vi "4_Generate_pulse_on_multiple channels.vi"() -> ()   [LabVIEW 2014]
uses:
  <vilib>/Swabian Instruments/Pulse Streamer/PulseStreamer/PulseStreamer/typedefs/typedef_TriggerStart.ctl
  <vilib>/Swabian Instruments/Pulse Streamer/PulseStreamer/PulsePattern/PulsePattern.lvclass
  <vilib>/Swabian Instruments/Pulse Streamer/PulseStreamer/typedefs/typedef_ChannelNumber.ctl
  <vilib>/Swabian Instruments/Pulse Streamer/PulseStreamer/Sequence/Sequence.lvclass
  <vilib>/Swabian Instruments/Pulse Streamer/PulseStreamer/PulseStreamer/stream/stream (Sequence).vi
  <vilib>/Swabian Instruments/Pulse Streamer/PulseStreamer/PulseStreamer/PulseStreamer.lvclass
  <vilib>/Swabian Instruments/Pulse Streamer/PulseStreamer/PulseStreamer.lvlib
panel:
  in  "nRuns":i64=1
  in  "ip or hostname":string="pulsestreamer"
  in  "Duration LOW":i64=1000
  out "error out":errorcluster
  in  "Repeat":u32=3
  in  "Start Type":T1
  in  "Duration HIGH":i64=500
  # "This example demonstrates how to generate synchronous signals on multiple channels.\n\nThe generated sequence consists of a square pulse on output channel \"0\" and three consecutive pulses on channels \"1\" and \"2\". \nThe pulses on channels \"1\" and \"2\" start on the falling edge of the pulse on channel \"0\".\n\nThis pulse sequence can be repeated finite or infinite number of times by specifying value of \"nRuns\".\nThe durations of each pulse are automatically split so that the Generated sequence has the Run Length Encoding (RLE)."
  # "PULSE DEFINITION"
  # "Every sequence has a repeat counter which can be used to repeat a\nsequence 'Repeat' times. \nIf there is only one sequence 'nRuns' from the 'stream' method should\nbe always used, because with 'Repeat' the data transferred to the \nPulsestreamer is repeated 'Repeat' times whereas nRuns sends the sequence\nonly once.\nRepeat >1 should be used when several sequences are combined and \neach sequence needs to be repeated."
  # "'nRuns' defines how many time the sequence has to be repeated by hardware\nnRuns<0 means that sequence will be repeated indefinitely"
  # "Defines whether the sequence starts \n* immediatly after it was uploaded  (IMMEDIATE)\n* after a software trigger (startNow) has been sent (SOFTWARE)\n* with an external trigger signal to \"Trigger\" input on the corresponding edge (HW_RISING, HW_FALLING, HW_RISING_AND_FALLING)."
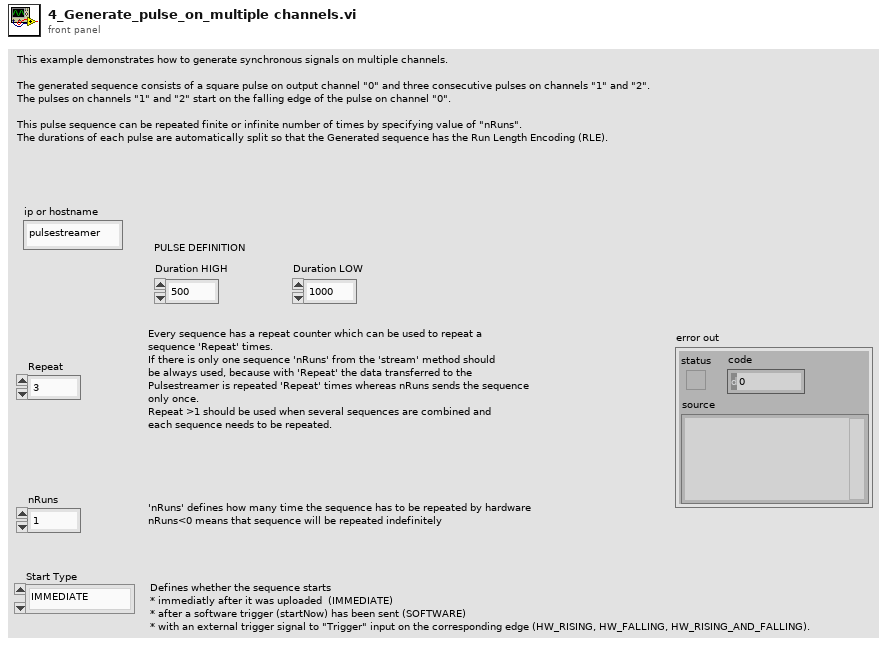
[diagram p1: front panel]
types:
  T1 = typedef "PulseStreamer.lvlib/PulseStreamer.lvclass/typedef_TriggerStart.ctl" = enum16{"IMMEDIATE", "SOFTWARE", "HW_RISING", "HW_FALLING", "HW_RISING_AND_FALLING"}
  T2 = typedef "PulseStreamer.lvlib/typedef_ChannelNumber.ctl" = i16
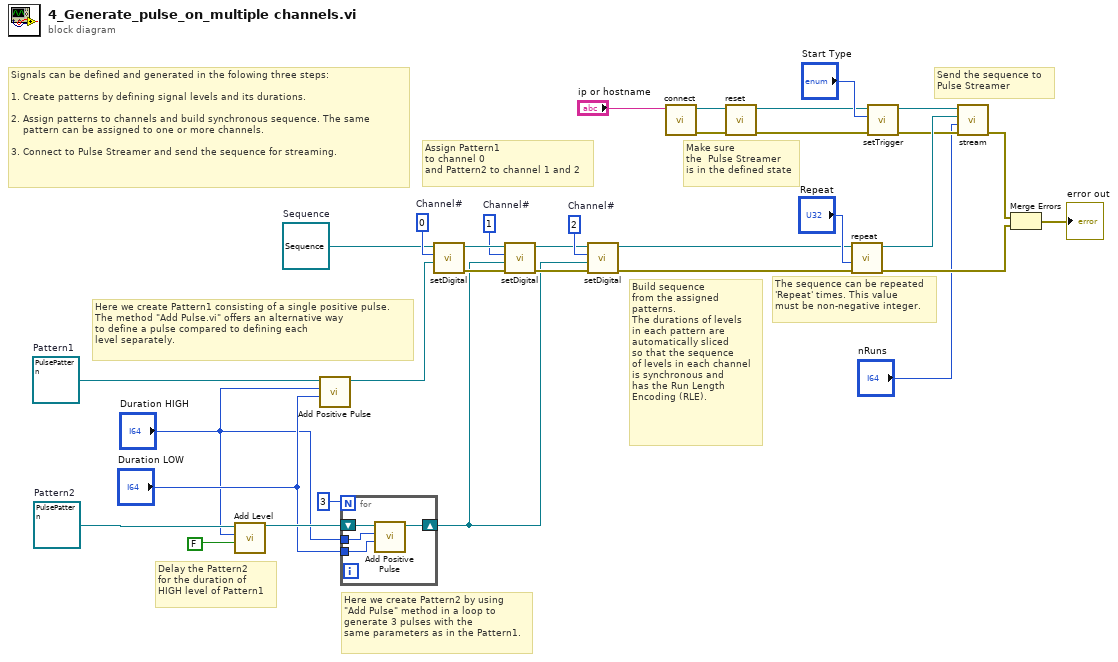
[diagram p0: block diagram]
diagram:
  w17 = T2 1  # Channel#
  w21 = T2 2  # Channel#
  w7 = refnum<class "PulsePattern.lvclass"> refnum  # Pattern2
  w23 = refnum<class "Sequence.lvclass"> refnum  # Sequence
  w27 = T2 0  # Channel#
  w13 = refnum<class "PulsePattern.lvclass"> refnum  # Pattern1
  # "Make sure\nthe  Pulse Streamer\nis in the defined state"
  # "Delay the Pattern2\nfor the duration of\nHIGH level of Pattern1"
  # "Here we create Pattern2 by using \n\"Add Pulse\" method in a loop to \ngenerate 3 pulses with the \nsame parameters as in the Pattern1."
  # "Send the sequence to \nPulse Streamer"
  # "Build sequence \nfrom the assigned \npatterns. \nThe durations of levels\nin each pattern are \nautomatically sliced \nso that the sequence \nof levels in each channel\nis synchronous and \nhas the Run Length \nEncoding (RLE)."
  # "The sequence can be repeated\n'Repeat' times. This value \nmust be non-negative integer."
  # "Assign Pattern1 \nto channel 0\nand Pattern2 to channel 1 and 2"
  # "Here we create Pattern1 consisting of a single positive pulse.\nThe method \"Add Pulse.vi\" offers an alternative way\nto define a pulse compared to defining each \nlevel separately."
  # "Signals can be defined and generated in the folowing three steps:\n\n1. Create patterns by defining signal levels and its durations.\n\n2. Assign patterns to channels and build synchronous sequence. The same\n    pattern can be assigned to one or more channels.\n\n3. Connect to Pulse Streamer and send the sequence for streaming."
  n1 = call <vilib>:"Add Level.vi"("Level"=FALSE, "Duration"="Duration HIGH", "Digital Sequence in"=w7) -> ("Digital Sequence out"=w6:refnum<class "PulsePattern.lvclass">)  [unwired: 8 in]
  n2 = call <vilib>:"Add Positive Pulse.vi"("Duration LOW"="Duration LOW", "Duration HIGH"="Duration HIGH", "Digital Pattern in"=w13) -> ("Digital Pattern out"=w14:refnum<class "PulsePattern.lvclass">)  [unwired: 8 in]
  n3 = for {
    N: 3 -> [_]
    shift-right: [w36] -> w8
    shift-left: w6 -> [w37]
    tunnel: "Duration HIGH" -> [w35]
    tunnel: "Duration LOW" -> [w34]
    n4 = call <vilib>:"Add Positive Pulse.vi"("Duration LOW"=w34, "Duration HIGH"=w35, "Digital Pattern in"=w37) -> ("Digital Pattern out"=w36:refnum<class "PulsePattern.lvclass">)  [unwired: 8 in]
  }
  n5 = call-dynamic "setDigital.vi"("PulsePattern"=w14, "channel"=w27, "Sequence in"=w23) -> ("error out"=w18:errorcluster, "Sequence out"=w19:refnum<class "Sequence.lvclass">)  [unwired: 7 in]
  n6 = call-dynamic "setDigital.vi"("error in (no error)"=w18, "PulsePattern"=w8, "channel"=w17, "Sequence in"=w19) -> ("error out"=w15:errorcluster, "Sequence out"=w16:refnum<class "Sequence.lvclass">)  [unwired: 6 in]
  n7 = call-dynamic "setDigital.vi"("error in (no error)"=w15, "PulsePattern"=w8, "channel"=w21, "Sequence in"=w16) -> ("error out"=w22:errorcluster, "Sequence out"=w3:refnum<class "Sequence.lvclass">)  [unwired: 6 in]
  n8 = call <vilib>:"connect.vi"("ip"="ip or hostname") -> ("error out"=w10:errorcluster, "Pulse Streamer out"=w12:refnum<class "PulseStreamer.lvclass">)  [unwired: 9 in]
  n9 = call <vilib>:"reset.vi"("error in (no error)"=w10, "Pulse Streamer in"=w12) -> ("error out"=w9:errorcluster, "Pulse Streamer out"=w11:refnum<class "PulseStreamer.lvclass">)  [unwired: 8 in]
  n10 = call <vilib>:"repeat.vi"("error in (no error)"=w22, "Repeat count"="Repeat", "Sequence in"=w3) -> ("error out"=w24:errorcluster, "Sequence out"=w33:refnum<class "Sequence.lvclass">)  [unwired: 7 in]
  n11 = call-dynamic "setTrigger.vi"("error in (no error)"=w9, "start"="Start Type", "Pulse Streamer in"=w11) -> ("error out"=w30:errorcluster, "Pulse Streamer out"=w31:refnum<class "PulseStreamer.lvclass">)  [unwired: 7 in]
  n12 = call-poly <vilib>:"stream.vi"("error in (no error)"=w30, "n_runs"="nRuns", "sequence"=w33, "Pulse Streamer in"=w31) -> ("error out"=w25:errorcluster)  [unwired: 4 in, 1 out]
  n13 = Merge Errors(w25, w24) -> (→"error out":errorcluster)
